vi "LoadWaveformSetupTrigger.vi"() -> ()   [LabVIEW 2012]
uses:
  Madlib.dll
panel:
  in  "Input Data Array":dbl[](array[numeric]) format="%.2f"
  in  "Axis":u32
  in  "DAC Rate (ms)  (time between steps)":dbl=0.0333333 min=0.0333333 max=5.0 format="%.4f"
  in  "Number of Position Values (steps)":u32=2 min=2 max=1000
  out "Return Code":string
  # "This example shows how to setup and trigger a position control waveform \nusing a two step process."
  # "X = 1\nY = 2\nZ = 3"
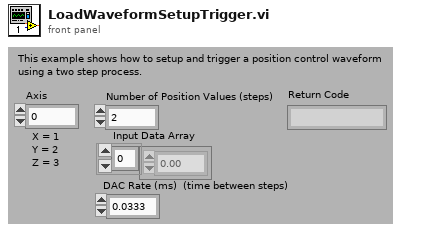
[diagram p1: front panel]
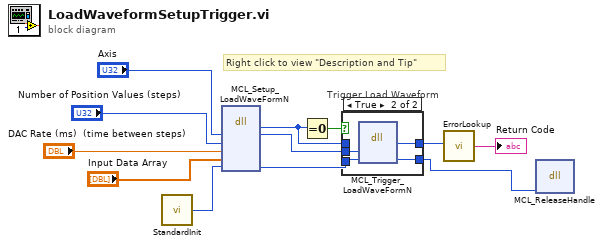
[diagram p0: block diagram]
diagram:
  # "Right click to view \"Description and Tip\""
  n1 = call "StandardInit.vi"() -> ("Outgoing Handle"=w4:i32)  [unwired: 1 in]
  n2 = dll-call lib="C:/Users/Labview/Desktop/SRR/Madlib_x64/Labview Examples/MADLib.dll" fn="MCL_Setup_LoadWaveFormN" label="Setup LoadWaveFormN"("axis"="Axis", "DataPoints"="Number of Position Values (steps)", "milliseconds"="DAC Rate (ms)  (time between steps)", "waveform"="Input Data Array", "handle"=w4) -> (w8:i32, "axis"=w9:u32, "handle"=w7:i32)  [unwired: 6 in, 2 out]
  n3 = Equal To 0?(x=w8) -> (x = 0?=w10:bool)
  n4 = case "Trigger Load Waveform" shown="True" w10 {
    tunnel: w9 -> [_ w18]
    tunnel: [w14 w17] -> w6
    tunnel: w8 -> [w14 _]
    tunnel: w7 -> [w13 w16]
    tunnel: [w13 w15] -> w5
    frame False {
    }
    frame True {
      n5 = dll-call lib="C:/Users/Labview/Desktop/SRR/Madlib_x64/Labview Examples/MADLib.dll" fn="MCL_Trigger_LoadWaveFormN" ("Trigger Load Waveform")("axis"=w18, "handle"=w16) -> (w17:i32, "handle"=w15:i32)  [unwired: 4 in, 2 out]
    }
  }
  n6 = call "ErrorLookup.vi"("Error Code"=w6) -> ("Error"=→"Return Code":string)
  n7 = dll-call lib="C:/Users/Labview/Desktop/SRR/Madlib_x64/Labview Examples/MADLib.dll" fn="MCL_ReleaseHandle"("handle"=w5) -> ()  [unwired: 5 in, 2 out]
